vi "det.vi"() -> ()   [LabVIEW 2011]
uses:
  <vilib>/express/express analysis/Spectral/Block/exnSpectralBlock spectral measurements RMS poly.vi
  <vilib>/express/express analysis/Spectral/Block/exnSpectralBlock spectral measurements RMS DDT.vi
  <vilib>/express/express analysis/Spectral/XNode/ExpressSpectralMeasurementsBlockNode.xnode
  <vilib>/measure/NI_MABase.lvlib
panel:
  out "Dynamic Data Type":dynamicdata(graph)
  out "size(s) 2":i32
  out "size(s)":i32
  in  "?":bool
  out "?":bool
  in  "Duration (s)":dbl(slide)=5.0 scale=0.05..1.0
  in  "?":bool
  out "?":bool
  out "?":bool
  in  "?":bool
  in  "?":dbl(slide)=100.0 min=50.0 max=1000.0 scale=50.0..5000.0
  out "DOLNA 2":dbl
  out "GÓRNA 2":dbl
  in  "?":dbl(knob)=100.0 min=50.0 max=10000.0 scale=50.0..10000.0
  out "?":dbl
  out "?":bool
  out "?":bool
  out "?":dbl
  out "?":dbl
  in  "częstotliwość środkowa":dbl(slide) min=0.0 max=20000.0 scale=50.0..20000.0
  in  "tolerancja":dbl(slide) min=0.0 max=1000.0 scale=0.0..1000.0
  out "?":bool
  in  "?":dbl(slide) scale=0.0..0.0005
  out "max value":dbl(slide) scale=0.0..0.0005
  out "?":bool
  out "?":bool
  out "?":bool
  out "?":bool
  in  "?":bool
  out "?":dbl
  out "Filtered Signal":dynamicdata(graph)
  out "?":bool
  out "?":bool
  in  "?":bool
  in  "?":dbl(slide)=100.0 min=50.0 max=1000.0 scale=50.0..10000.0
  in  "?":bool
  in  "?":bool
  in  "Lower Cut-Off":dbl(knob)=100.0 min=50.0 max=10000.0 scale=40.0..10000.0
  out "Lower Cut-Off":dbl=100.0
  out "DOLNA":dbl
  out "GÓRNA":dbl
  in  "?":dbl(knob)=100.0 min=50.0 max=10000.0 scale=50.0..10000.0
  in  "symulowana fgen":dbl(knob)=500.0 caption="Frequency" min=50.0 max=10000.0 scale=50.0..10000.0
  in  "?":bool
  out "?":dynamicdata(graph)
  # "DŹWIĘK ON/OFF"
  # "WYBÓR DETEKCJI"
  # "POZIOM SYGNAŁU"
  # "CZĘSTOTLIWOŚĆ"
  # "ON"
  # "S"
  # "POZIOM"
  # "OFF"
  # "U"
  # "U > S?"
  # "L"
  # "S > L?"
  # "WYBÓR ŹRÓDŁA"
  # "SYMULACJA"
  # "WEJŚCIE LINIOWE"
  # "GŁÓWNA CZĘSTOTLIWOŚĆ\nSYGNAL SUROWY"
  # "CZĘSTOTLIWOŚCI\n(BANDPASS)"
  # "bandwidth"
  # "CZĘSTOTLIWOŚĆ \n(LOWPASS)"
  # "CZĘSTOTLIWOŚCI\n(BANDSTOP)"
  # "bandwidth"
  # "czas próbki"
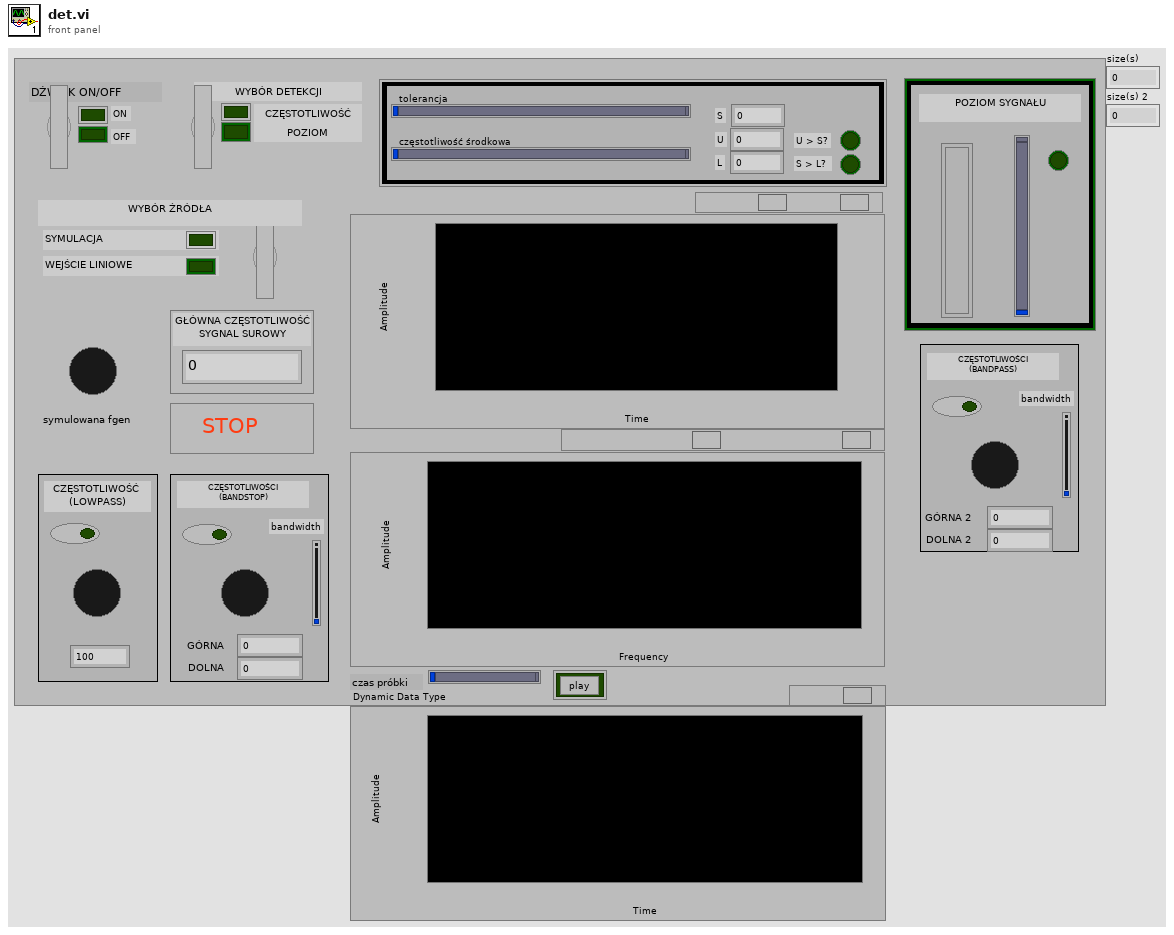
[diagram p1: front panel]
types:
  T1 = cluster{"averaging mode":u16, "weighting mode":u16, "number of averages":u32}
  T2 = cluster{"dB On (F)":bool, "unwrap phase (F)":bool, "convert to degree (F)":bool}
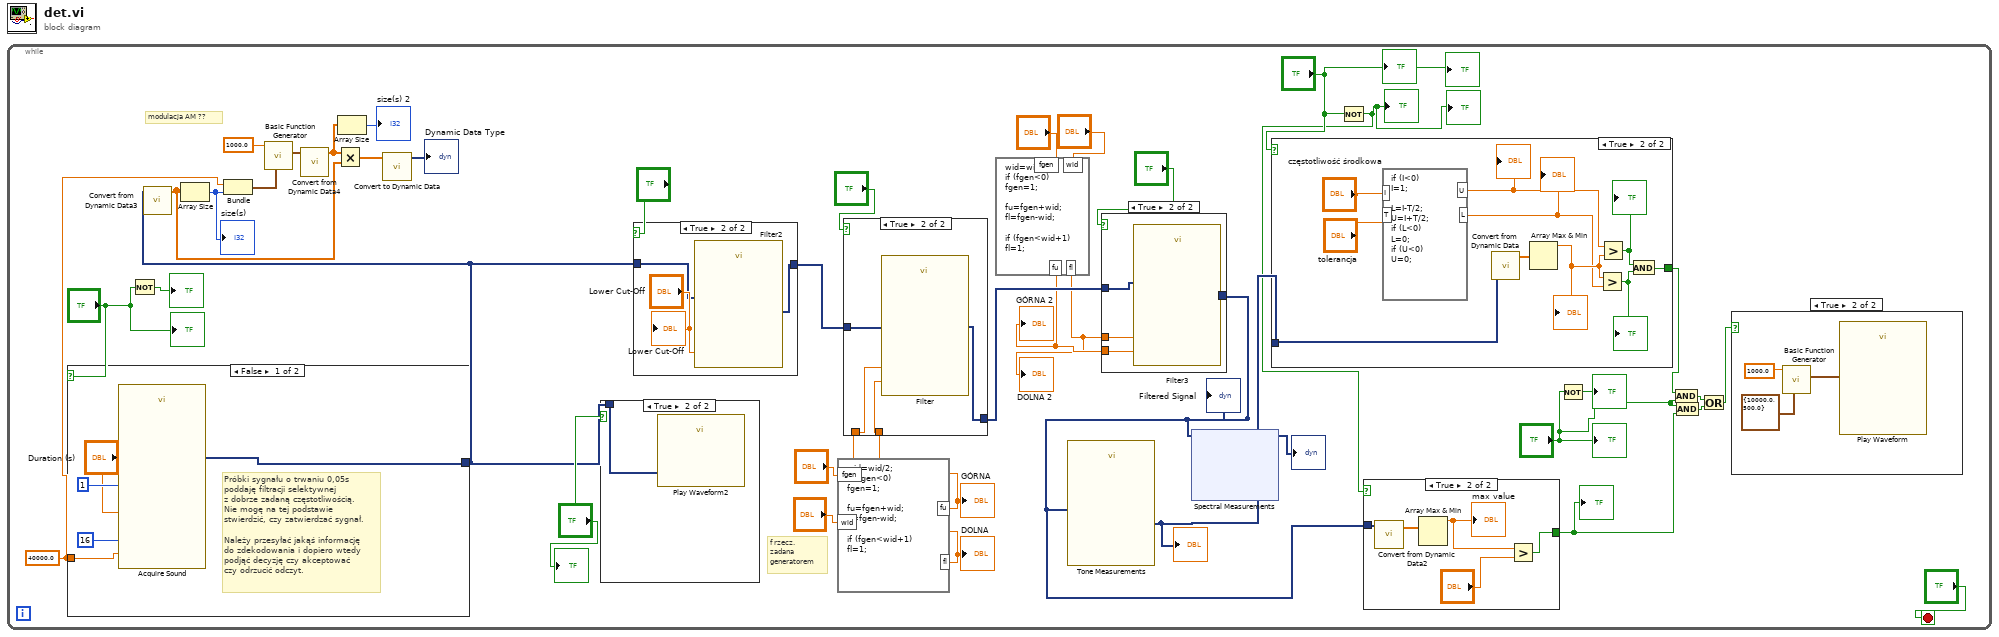
[diagram p0: block diagram]
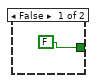
[diagram p3: hidden frame]
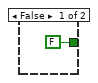
[diagram p6: hidden frame]
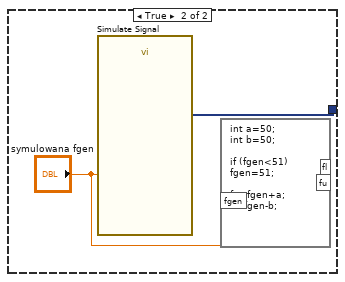
[diagram p9: hidden frame]
diagram:
  n1 = while {
    stop <- "?" stop-if-true
    w8 = 40000.0 ("Sample rate (")
    # "modulacja AM ??"
    # "f rzecz.\nzadana \ngeneratorem"
    n2 = case shown="False" "?" {
      tunnel: [w78 w81] -> w10
      tunnel: w8 -> [w76 _]
      frame False {
        # "Próbki sygnału o trwaniu 0,05s \npoddaję filtracji selektywnej\nz dobrze zadaną częstotliwością.\nNie mogę na tej podstawie\nstwierdzić, czy zatwierdzać sygnał.\n\nNależy przesyłać jakąś informację\ndo zdekodowania i dopiero wtedy\npodjąć decyzję czy akceptować\nczy odrzucić odczyt."
        n3 = call "Acquire Sound"("Duration (s)"="Duration (s)", "Sample rate (Hz)"=w76, "#Channels"=1, "Resolution (bits)"=16) -> ("Data"=w78:dynamicdata)  [unwired: 14 in, 1 out]
      }
      frame True {
        n4 = call "Simulate Signal"("Frequency"="symulowana fgen") -> ("Sine"=w81:dynamicdata)  [unwired: 13 in, 1 out]
        n5 = formula code="int a=50;\nint b=50;\n\nif (fgen<51)\nfgen=51;\n\nfu=fgen+a;\nfl=fgen-b;"("fgen"="symulowana fgen") -> ()  [unwired: 2 out]
      }
    }
    n6 = Not(x="?") -> (.not. x?=→"?":bool)
    n7 = call "Convert from Dynamic Data3"("Dynamic Data Type"=w10) -> ("Array"=w3:dbl[])  [unwired: 3 in]
    n8 = Array Size(array=w3) -> (size(s)=w9:i32)
    "size(s)" <- w9
    n9 = Bundle("Sample rate ("=w8, w9) -> (w7:cluster{"Sample rate (":dbl, i32})  [unwired: 1 in]
    n10 = call <vilib>:"Basic Function Generator.vi"("sampling info"=w7, "frequency"=1000.0) -> ("signal out"=w6:waveform(dbl))  [unwired: 7 in, 2 out]
    n11 = call "Convert from Dynamic Data4"("Dynamic Data Type"=w6) -> ("Array"=w4:dbl[])  [unwired: 3 in]
    n12 = Multiply(x=w4, y=w3) -> (x*y=w2:dbl[])
    n13 = Array Size(array=w4) -> (size(s)=→"size(s) 2":i32)
    n14 = call "Convert to Dynamic Data"("Array"=w2) -> ("Dynamic Data Type"=→"Dynamic Data Type":dynamicdata)  [unwired: 3 in]
    n15 = case shown="True" "?" {
      tunnel: w10 -> [_ w41]
      frame False {
      }
      frame True {
        n16 = call "Play Waveform2"("Data"=w41) -> ()  [unwired: 18 in, 1 out]
      }
    }
    n17 = case shown="True" "?" {
      tunnel: w10 -> [w67 w69]
      tunnel: [w67 w68] -> w37
      frame False {
      }
      frame True {
        n18 = call "Filter2"("Lower Cut-Off"="Lower Cut-Off", "Signal"=w69) -> ("Filtered Signal"=w68:dynamicdata)  [unwired: 8 in, 1 out]
        "Lower Cut-Off" <- "Lower Cut-Off"
      }
    }
    n19 = formula code="wid=wid/2;\nif (fgen<0)\nfgen=1;\n\nfu=fgen+wid;\nfl=fgen-wid;\n\nif (fgen<wid+1)\nfl=1;"("fgen"="?", "wid"="?") -> ("fl"=w25:dbl, "fu"=w24:dbl)
    "GÓRNA" <- w24
    "DOLNA" <- w25
    n20 = case shown="True" "?" {
      tunnel: w25 -> [_ w72]
      tunnel: w24 -> [_ w73]
      tunnel: w37 -> [w71 w75]
      tunnel: [w71 w74] -> w33
      frame False {
      }
      frame True {
        n21 = call "Filter"("Lower Cut-Off"=w72, "Upper Cut-Off"=w73, "Signal"=w75) -> ("Filtered Signal"=w74:dynamicdata)  [unwired: 7 in, 1 out]
      }
    }
    n22 = formula code="wid=wid/2;\nif (fgen<0)\nfgen=1;\n\nfu=fgen+wid;\nfl=fgen-wid;\n\nif (fgen<wid+1)\nfl=1;"("fgen"="?", "wid"="?") -> ("fu"=w32:dbl, "fl"=w31:dbl)
    "DOLNA 2" <- w31
    "GÓRNA 2" <- w32
    n23 = case shown="True" "?" {
      tunnel: w32 -> [_ w55]
      tunnel: w31 -> [_ w54]
      tunnel: w33 -> [w51 w53]
      tunnel: [w51 w52] -> w13
      frame False {
      }
      frame True {
        n24 = call "Filter3"("Lower Cut-Off"=w54, "Upper Cut-Off"=w55, "Signal"=w53) -> ("Filtered Signal"=w52:dynamicdata)  [unwired: 7 in, 1 out]
      }
    }
    "Filtered Signal" <- w13
    n25 = call "Tone Measurements"("Signals"=w13) -> ("Frequency"=w34:dynamicdata)  [unwired: 9 in, 1 out]
    "?" <- w34
    n26 = xnode "Spectral Measurements"("Signals"=w13) -> ("FFT - (RMS)"=→"?":dynamicdata)  [unwired: 1 in, 2 out]
    n27 = case shown="True" "?" {
      tunnel: w34 -> [_ w58]
      tunnel: [FALSE w57] -> w23
      frame False {
      }
      frame True {
        n28 = formula code="if (I<0)\nI=1;\n\nL=I-T/2;\nU=I+T/2;\nif (L<0)\nL=0;\nif (U<0)\nU=0;"("T"="tolerancja", "I"="częstotliwość środkowa") -> ("U"=w61:dbl, "L"=w62:dbl)
        "?" <- w61
        "?" <- w62
        n29 = call "Convert from Dynamic Data"("Dynamic Data Type"=w58) -> ("Array"=w66:dbl[])  [unwired: 3 in]
        n30 = Array Max & Min(array=w66) -> (max value=w65:dbl)  [unwired: 3 out]
        "?" <- w65
        n31 = Greater?(x=w65, y=w62) -> (0:w64:bool)
        "?" <- w64
        n32 = Greater?(x=w61, y=w65) -> (0:w63:bool)
        "?" <- w63
        n33 = And(x=w63, y=w64) -> (x .and. y?=w57:bool)
      }
    }
    n34 = Not(x="?") -> (.not. x?=w16:bool)
    "?" <- w16
    "?" <- w16
    n35 = case shown="True" w16 {
      tunnel: [FALSE w46] -> w15
      tunnel: w13 -> [_ w43]
      frame False {
      }
      frame True {
        n36 = call "Convert from Dynamic Data2"("Dynamic Data Type"=w43) -> ("Array"=w47:dbl[])  [unwired: 3 in]
        n37 = Array Max & Min(array=w47) -> (max value=w44:dbl)  [unwired: 3 out]
        "max value" <- w44
        n38 = Greater?(x=w44, y="?") -> (0:w46:bool)
      }
    }
    "?" <- w15
    n39 = Not(x="?") -> (.not. x?=→"?":bool)
    n40 = And(x=w23, y="?") -> (x .and. y?=w22:bool)
    n41 = And(x="?", y=w15) -> (x .and. y?=w21:bool)
    n42 = Or(x=w22, y=w21) -> (x .or. y?=w20:bool)
    n43 = case shown="True" w20 {
      frame False {
      }
      frame True {
        n44 = call <vilib>:"Basic Function Generator.vi"("sampling info"=cluster{"Fs":dbl, "#s":dbl} {"Fs"=10000.0, "#s"=500.0}, "frequency"=1000.0) -> ("signal out"=w50:waveform(dbl))  [unwired: 7 in, 2 out]
        n45 = call "Play Waveform"("Data"=w50) -> ()  [unwired: 18 in, 1 out]
      }
    }
    "?" <- "?"
    "?" <- "?"
    "?" <- "?"
    "?" <- "?"
    "?" <- "?"
  }
